vi "Main Control.vi"() -> ()   [LabVIEW 2016]
doc: "Read 4 Atlas Scientific sensors : Temperature, Oxygen, pH, Conductivity. First detects the presence of sensors and theis USB port, then reads them with the set sampling rate"
panel:
  in  "Cond On?":bool=TRUE
  in  "pH On?":bool=TRUE
  in  "Oxygen On?":bool=TRUE
  in  "Temp On?":bool=TRUE
  out "Graphe déroulant":T1(graph)={"Temp"=0.0, "Humid"=0.0, "Lum"=31.283, "Force"=0.0}
  out "refnum file out":refnum<file>
  in  "Start saving":bool
  in  "stop":bool
  out "Status":string
  in  "Sampling rate (s)":u16=2 min=2
  # "ATLAS SCIENTIFIC\nSENSORS ACQUISITION"
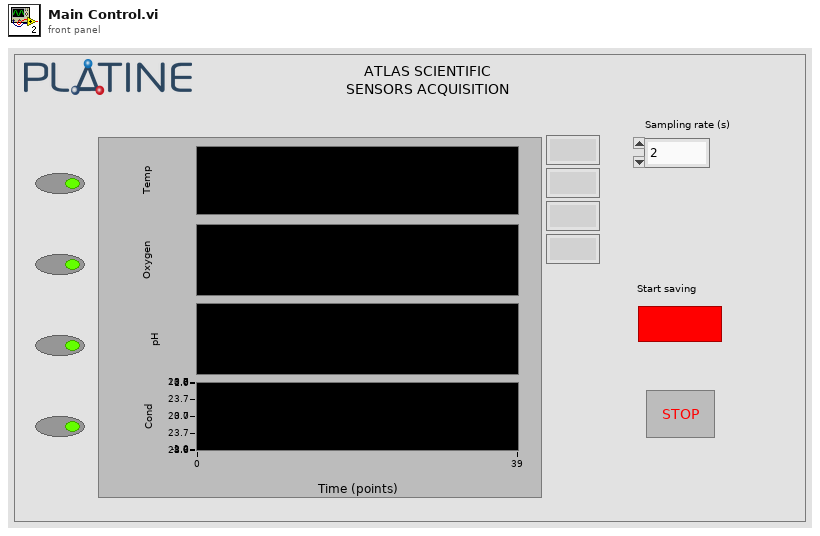
[diagram p1: front panel]
types:
  T1 = cluster{"Temp":dbl, "Humid":dbl, "Lum":dbl, "Force":dbl}
  T2 = cluster{"Temp":dbl, "Humid":dbl, "Lum":dbl, "Force":dbl}[]
  T3 = typedef "Visa com cluster def (subVI).ctl" = cluster{"Sensor":string, "VISA resource name":refnum<visa-resource-name>, "error in/out":errorcluster, "bytes read":u32, "Com found ?":bool}
  T4 = enum16{"open", "replace", "create", "open or create", "replace or create", "replace or create with confirmation"}
  T5 = cluster{"Reading":dbl, "Reading":dbl, "Reading":dbl, "Reading":dbl}
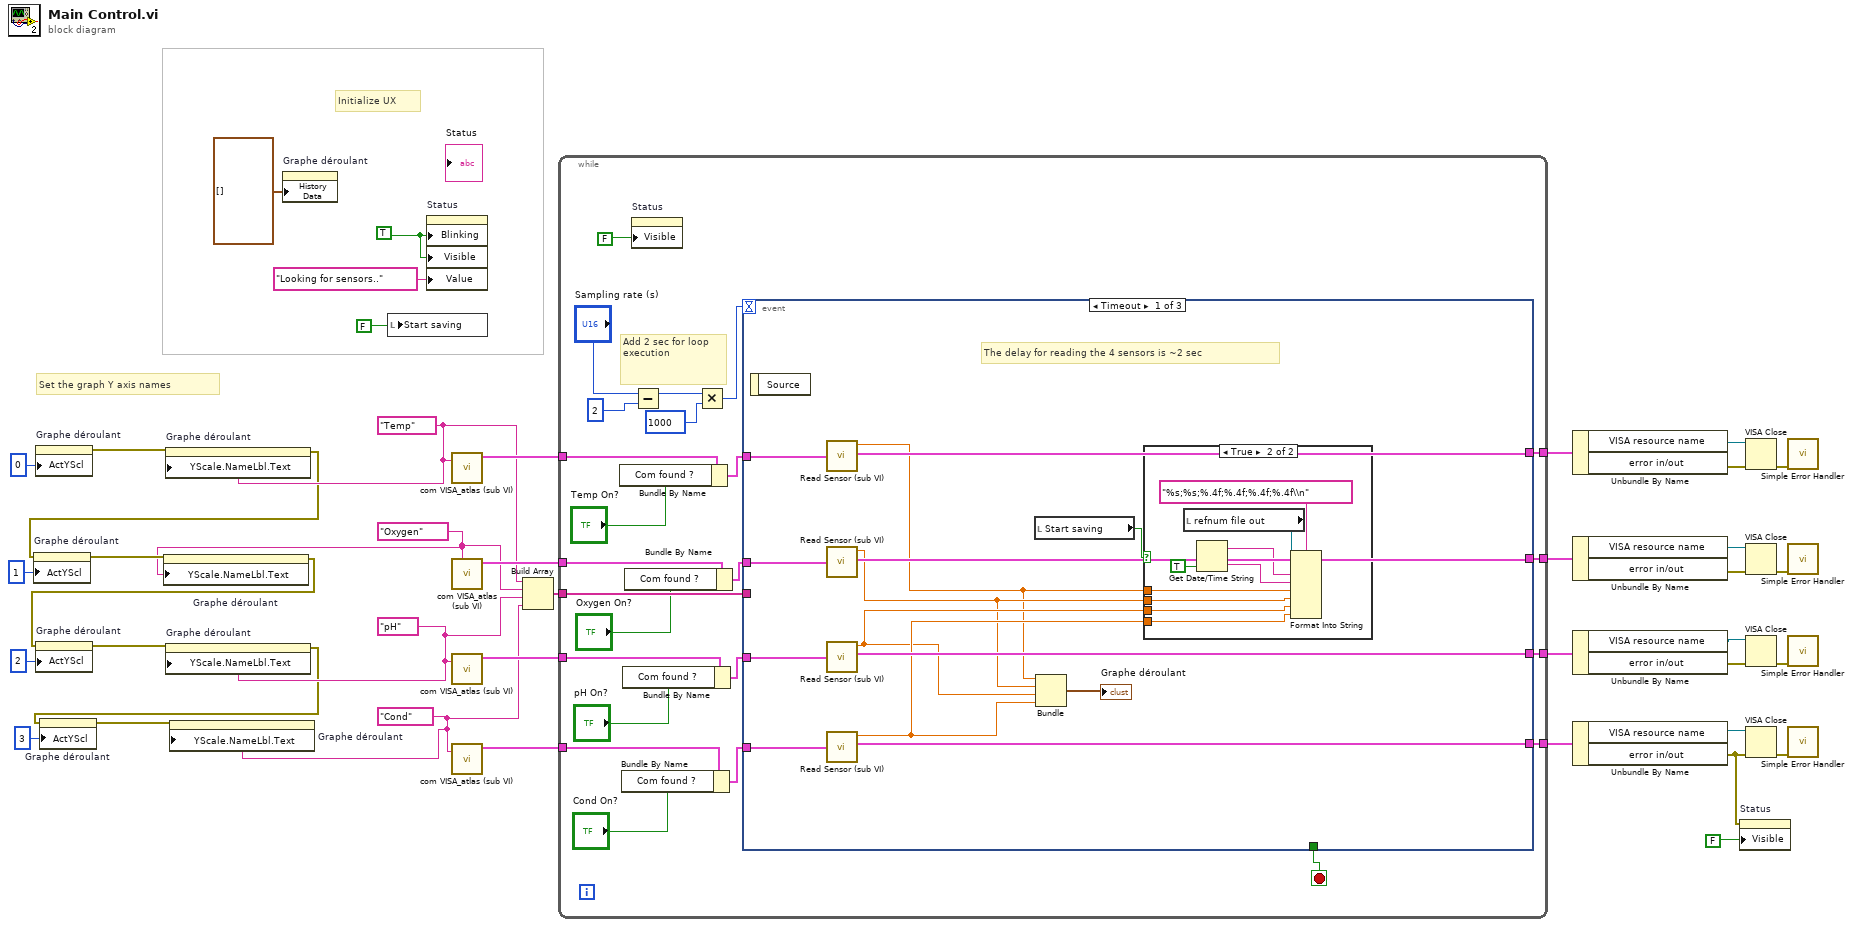
[diagram p0: block diagram]
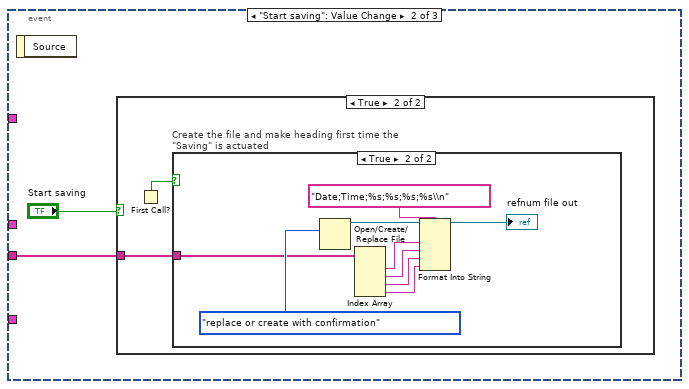
[diagram p3: hidden frame]
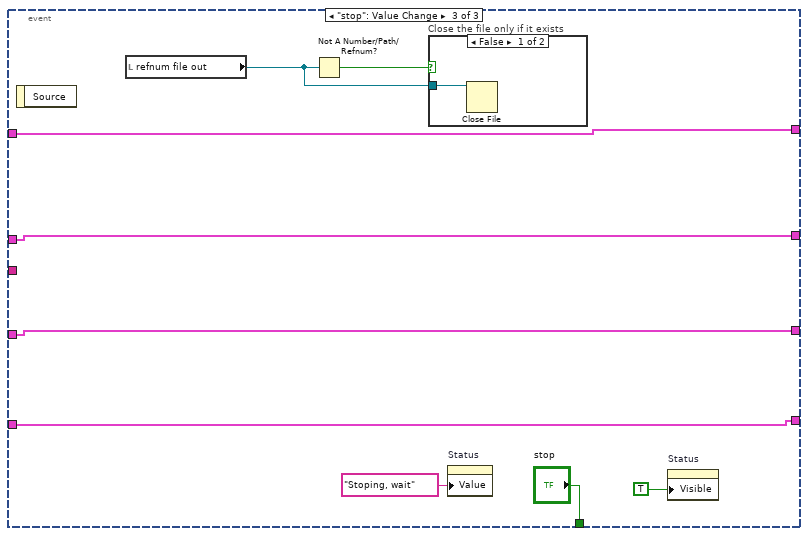
[diagram p6: hidden frame]
diagram:
  w22 = TRUE ("Blinking")
  w17 = "Temp" ("Combo Box")
  w8 = "Oxygen" ("Combo Box")
  w10 = "pH" ("Combo Box")
  w9 = "Cond" ("Combo Box")
  # "Initialize UX"
  # "Set the graph Y axis names"
  n1 = property on="Graphe déroulant" class="WFChart (strict)"("ActYScl"=0 ("Active Y Scale")) -> (error out=w18:errorcluster)  [unwired: 2 in, 1 out]
  n2 = property on="Graphe déroulant" class="WFChart (strict)"(error in=w18, "YScale.NameLbl.Text"=w17) -> (error out=w7:errorcluster)  [unwired: 1 in, 1 out]
  n3 = property on="Graphe déroulant" class="WFChart (strict)"(error in=w7, "ActYScl"=1 ("Active Y Scale")) -> (error out=w15:errorcluster)  [unwired: 1 in, 1 out]
  n4 = property on="Graphe déroulant" class="WFChart (strict)"(error in=w15, "YScale.NameLbl.Text"=w8) -> (error out=w6:errorcluster)  [unwired: 1 in, 1 out]
  n5 = property on="Graphe déroulant" class="WFChart (strict)"(error in=w6, "ActYScl"=2 ("Active Y Scale")) -> (error out=w13:errorcluster)  [unwired: 1 in, 1 out]
  n6 = property on="Graphe déroulant" class="WFChart (strict)"(error in=w13, "YScale.NameLbl.Text"=w10) -> (error out=w5:errorcluster)  [unwired: 1 in, 1 out]
  n7 = property on="Graphe déroulant" class="WFChart (strict)"(error in=w5, "ActYScl"=3 ("Active Y Scale")) -> (error out=w11:errorcluster)  [unwired: 1 in, 1 out]
  n8 = property on="Graphe déroulant" class="WFChart (strict)"(error in=w11, "YScale.NameLbl.Text"=w9) -> ()  [unwired: 1 in, 2 out]
  n9 = property on="Graphe déroulant" class="WFChart (strict)"("History Data"=T2 []) -> ()  [unwired: 2 in, 2 out]
  n10 = local write "Start saving"(FALSE ("Start saving")) -> ()
  n11 = property on="Status" class="Str"("Blinking"=w22, "Visible"=w22, "Value"="Looking for sensors.." ("Status")) -> ()  [unwired: 2 in, 2 out]
  n12 = call "com VISA_atlas (sub VI).vi"("Sensor"=w17) -> ("Output cluster"=w24:T3)  [unwired: 3 in, 1 out]
  n13 = call "com VISA_atlas (sub VI).vi"("Sensor"=w8) -> ("Output cluster"=w32:T3)  [unwired: 3 in, 1 out]
  n14 = call "com VISA_atlas (sub VI).vi"("Sensor"=w10) -> ("Output cluster"=w37:T3)  [unwired: 3 in, 1 out]
  n15 = call "com VISA_atlas (sub VI).vi"("Sensor"=w9) -> ("Output cluster"=w40:T3)  [unwired: 3 in, 1 out]
  n16 = Build Array(w17, w8, w10, w9) -> (w21:string[])
  n17 = while {
    tunnel: w40 -> [w43]
    tunnel: [w64] -> w39
    tunnel: w37 -> [w46]
    tunnel: [w63] -> w33
    tunnel: w32 -> [w49]
    tunnel: [w62] -> w28
    tunnel: w24 -> [w53]
    tunnel: [w61] -> w23
    tunnel: w21 -> [w56]
    stop <- w65 stop-if-true
    # "Add 2 sec for loop execution"
    n18 = Bundle By Name(cluster=w53, "Com found ?"="Temp On?") -> (w51:T3)
    n19 = Bundle By Name(cluster=w43, "Com found ?"="Cond On?") -> (w42:T3)
    n20 = Bundle By Name(cluster=w46, "Com found ?"="pH On?") -> (w45:T3)
    n21 = Bundle By Name(cluster=w49, "Com found ?"="Oxygen On?") -> (w48:T3)
    n22 = property on="Status" class="Str"("Visible"=FALSE) -> ()  [unwired: 2 in, 2 out]
    n23 = Subtract(x="Sampling rate (s)", y=u16 2) -> (x-y=w55:u16)
    n24 = Multiply(x=w55, y=u16 1000 ("x")) -> (x*y=w60:u16)
    n25 = event shown="[0] Timeout" {
      selector: _ -> [_ _ _]
      dyn-events: _ -> [_ _ _]
      timeout: w60 -> [_ _ _]
      tunnel: [_ _ "stop"] -> w65
      tunnel: w42 -> [w79 _ w102]
      tunnel: [w78 _ w102] -> w64
      tunnel: w45 -> [w77 _ w103]
      tunnel: [w76 _ w103] -> w63
      tunnel: w48 -> [w75 _ w104]
      tunnel: [w74 _ w104] -> w62
      tunnel: w51 -> [w73 _ w105]
      tunnel: [w72 _ w105] -> w61
      tunnel: w56 -> [_ w89 _]
      event Timeout {
        # "The delay for reading the 4 sensors is ~2 sec"
        n26 = event-data() -> ()  [unwired: 1 in, 1 out]
        n27 = call "Read Sensor (sub VI).vi"("Input cluster"=w73) -> ("Reading"=w66:dbl, "Output cluster"=w72:T3)  [unwired: 2 in]
        n28 = call "Read Sensor (sub VI).vi"("Input cluster"=w75) -> ("Reading"=w67:dbl, "Output cluster"=w74:T3)  [unwired: 2 in]
        n29 = call "Read Sensor (sub VI).vi"("Input cluster"=w77) -> ("Reading"=w68:dbl, "Output cluster"=w76:T3)  [unwired: 2 in]
        n30 = call "Read Sensor (sub VI).vi"("Input cluster"=w79) -> ("Reading"=w69:dbl, "Output cluster"=w78:T3)  [unwired: 2 in]
        n31 = local read "Start saving"() -> (w71:bool)
        n32 = Bundle("Reading"=w66, "Reading"=w67, "Reading"=w68, "Reading"=w69) -> (→"Graphe déroulant":T5)  [unwired: 1 in]
        n33 = case shown="True" w71 {
          tunnel: w66 -> [_ w83]
          tunnel: w67 -> [_ w82]
          tunnel: w68 -> [_ w81]
          tunnel: w69 -> [_ w80]
          frame False {
          }
          frame True {
            n34 = local read "refnum file out"() -> (w88:refnum<file>)
            n35 = Get Date/Time String(want seconds? (F)=TRUE) -> (date string=w85:string, time string=w84:string)  [unwired: 2 in]
            n36 = Format Into String(format string="%s;%s;%.4f;%.4f;%.4f;%.4f\\n", initial string=w88, w85, w84, w83, w82, w81, w80) -> ()  [unwired: 1 in, 2 out]
          }
        }
      }
      event "Start saving": Value Change {
        n37 = event-data() -> ()  [unwired: 1 in, 1 out]
        n38 = case shown="True" "Start saving" {
          tunnel: w89 -> [_ w91]
          frame False {
          }
          frame True {
            n39 = First Call?() -> (First Call?: T/F=w92:bool)
            n40 = case "Create the file and make heading first time the \"Saving\" is actuated" shown="True" w92 {
              tunnel: w91 -> [_ w97]
              frame False {
              }
              frame True {
                n41 = Open/Create/Replace File(operation (0:open)=T4."replace or create with confirmation" ("opération (0 : open)")) -> (refnum out=w99:refnum<file>)  [unwired: 5 in, 2 out]
                n42 = Index Array(array=w97) -> (element #1=w96:string, element #2=w95:string, element #3=w94:string, element #4=w93:string)  [unwired: 4 in]
                n43 = Format Into String(format string="Date;Time;%s;%s;%s;%s\\n", initial string=w99, w96, w95, w94, w93) -> (resulting string=→"refnum file out":refnum<file>)  [unwired: 1 in, 1 out]
              }
            }
          }
        }
      }
      event "stop": Value Change {
        n44 = event-data() -> ()  [unwired: 1 in, 1 out]
        n45 = local read "refnum file out"() -> (w108:refnum<file>)
        n46 = Not A Number/Path/Refnum?(number/path/refnum=w108) -> (NaN/Path/Refnum?=w109:bool)
        n47 = case "Close the file only if it exists" shown="False" w109 {
          tunnel: w108 -> [w111 _]
          frame False {
            n48 = Close File(refnum=w111) -> ()  [unwired: 1 in, 2 out]
          }
          frame True {
          }
        }
        n49 = property on="Status" class="Str"("Value"="Stoping, wait" ("Status")) -> ()  [unwired: 2 in, 2 out]
        n50 = property on="Status" class="Str"("Visible"=TRUE ("Blinking")) -> ()  [unwired: 2 in, 2 out]
      }
    }
  }
  n51 = Unbundle By Name(w23) -> ("VISA resource name"=w26:refnum<visa-resource-name>, "error in/out"=w25:errorcluster)
  n52 = Unbundle By Name(w28) -> ("VISA resource name"=w30:refnum<visa-resource-name>, "error in/out"=w29:errorcluster)
  n53 = Unbundle By Name(w33) -> ("VISA resource name"=w35:refnum<visa-resource-name>, "error in/out"=w34:errorcluster)
  n54 = Unbundle By Name(w39) -> ("VISA resource name"=w38:refnum<visa-resource-name>, "error in/out"=w2:errorcluster)
  n55 = property on="Status" class="Str"(error in=w2, "Visible"=FALSE) -> ()  [unwired: 1 in, 2 out]
  n56 = VISA Close(VISA resource name=w26, error in (no error)=w25) -> (error out=w27:errorcluster)
  n57 = VISA Close(VISA resource name=w30, error in (no error)=w29) -> (error out=w31:errorcluster)
  n58 = VISA Close(VISA resource name=w35, error in (no error)=w34) -> (error out=w36:errorcluster)
  n59 = VISA Close(VISA resource name=w38, error in (no error)=w2) -> (error out=w41:errorcluster)
  n60 = call <vilib>:"Simple Error Handler.vi"("error in (no error)"=w27) -> ()  [unwired: 1 in, 8 out]
  n61 = call <vilib>:"Simple Error Handler.vi"("error in (no error)"=w31) -> ()  [unwired: 1 in, 8 out]
  n62 = call <vilib>:"Simple Error Handler.vi"("error in (no error)"=w36) -> ()  [unwired: 1 in, 8 out]
  n63 = call <vilib>:"Simple Error Handler.vi"("error in (no error)"=w41) -> ()  [unwired: 1 in, 8 out]
